vi "VI, Grow Panel Width to Control.vi"(5 "margin (20)":i32=20, 6 "error in":errorcluster, 8 "Ctl ref":refnum<vi>, 9 "VI ref":refnum<vi>) -> (0 "error out":errorcluster, 2 "Ctl ref dup":refnum<vi>, 3 "VI ref dup":refnum<vi>)   [LabVIEW 2010]
doc: "This function increases a panels width to display a control."
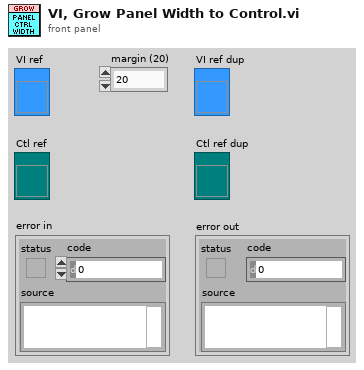
[diagram p1: front panel]
types:
  T1 = typedef "LVRectTypeDef.ctl" = cluster{"left":i16, "top":i16, "right":i16, "bottom":i16}
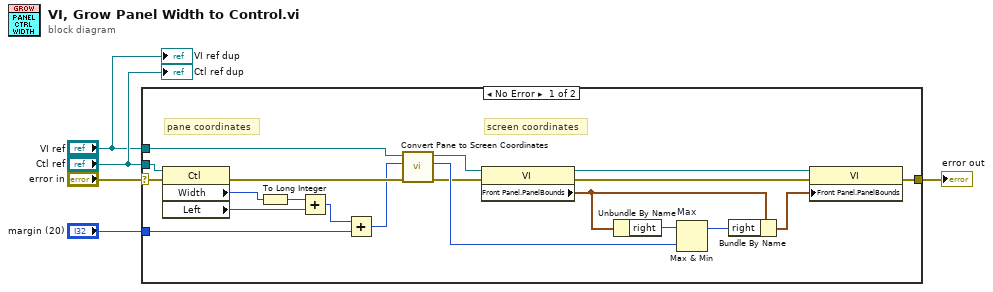
[diagram p0: block diagram]
diagram:
  n1 = case shown="No Error" "error in" {
    selector: "error in" -> [w24 w26]
    tunnel: [w21 w26] -> w5
    tunnel: "Ctl ref" -> [w25 _]
    tunnel: "VI ref" -> [w6 _]
    tunnel: "margin (20)" -> [w23 _]
    frame No Error {
      # "screen coordinates"
      # "pane coordinates"
      n2 = property class="Ctl"(reference=w25, error in=w24) -> (error out=w15:errorcluster, "Width"=w22:u32, "Left"=w14:i32)  [unwired: 1 out]
      n3 = To Long Integer(number=w22) -> (32bit integer=w18:i32)
      n4 = Add(x=w18, y=w14) -> (x+y=w17:i32)
      n5 = Add(x=w17, y=w23) -> (x+y=w13:i32)
      n6 = call "Convert Pane to Screen Coordinates.vi"("error in"=w15, "Horizontal"=w13, "VI ref"=w6) -> ("error out"=w11:errorcluster, "Horizontal out"=w12:i16, "VI ref dup"=w7:refnum<vi>)  [unwired: 3 in, 1 out]
      n7 = property class="VI"(reference=w7, error in=w11) -> (reference out=w8:refnum<vi>, error out=w10:errorcluster, "Front Panel.PanelBounds"=w9:T1)
      n8 = Unbundle By Name(w9) -> ("right"=w19:i16)
      n9 = Max & Min "Max"(x=w19, y=w12) -> (max(x,y)=w16:i16)  [unwired: 1 out]
      n10 = Bundle By Name(cluster=w9, "right"=w16) -> (w20:T1)
      n11 = property class="VI"(reference=w8, error in=w10, "Front Panel.PanelBounds"=w20) -> (error out=w21:errorcluster)  [unwired: 1 out]
    }
    frame Error {
    }
  }
  "error out" <- w5
  "VI ref dup" <- "VI ref"
  "Ctl ref dup" <- "Ctl ref"
